vi "PID Autotune Y-Axis.vi"() -> ()   [LabVIEW 2017]
uses:
  <vilib>/addons/control/pid/autopid.llb/PID autotuning parameters (adv).ctl
  <vilib>/myRIO/Common/Instrument Driver Framework/myRIO v1.0/UART/vis/myRIO v1.0 Close UART.vi
  <vilib>/addons/control/pid/pid.llb/PID Control Input Filter (DBL).vi
  <vilib>/myRIO/Common/Instrument Driver Framework/Utilities/vis/FPGA Ref Manager.vi
  <vilib>/myRIO/Common/Instrument Driver Framework/myRIO v1.0/myRIO v1.0 Reset FPGA.vi
  <vilib>/myRIO/Common/Instrument Driver Framework/myRIO v1.0/IRQ/vis/myRIO v1.0 IRQ Info FGV.vi
  <vilib>/myRIO/Common/Instrument Driver Framework/myRIO v1.0/IRQ/vis/myRIO v1.0 Timer IRQ Info FGV.vi
  <vilib>/myRIO/Common/Instrument Driver Framework/myRIO v1.0/IRQ/vis/myRIO v1.0 ISR Agent.vi
  <vilib>/myRIO/Instrument Drivers/Utilities/Utilities.lvlib
  <vilib>/addons/control/pid/NI_PID_pid.lvlib
  <vilib>/addons/control/pid/NI_PID_autopid.lvlib
  <vilib>/ptbypt/NI_PtbyPt.lvlib
panel:
  in  "alpha":dbl=0.1 format="%.2f"
  in  "gamma":dbl format="%.2f"
  in  "autotuning parameters":T1={"technique"=2, "type of controller"=1, "control specification"=0, "amplitude"=1.0} {"amplitude" format="%.2f"; "control specification" items=["normal", "fast", "slow"]; "type of controller" items=["P", "PI", "PID"]; "technique" items=["Step Open Loop", "Step Closed Loop", "Relay", "PID Relay"]}
  in  "reinitialize? (F)":bool
  out "tuning completed?":bool
  in  "auto? (F)":bool
  out "tuned PID gains":T2={"proportional gain (Kc)"=1.0, "integral time (Ti, min)"=0.01, "derivative time (Td, min)"=0.0} {"derivative time (Td, min)" format="%#.6g"; "integral time (Ti, min)" format="%#.6g"; "proportional gain (Kc)" format="%#.6g"}
  in  "autotune? (F)":bool
  out "Sensor Output":cluster{dbl, "output":dbl}(graph)
  out "Motion Data":T3
  in  "FWD/RVS":bool
  out "Time (s)":dbl
  out "Output String":string
  out "PID Output":dbl(graph)
  out "SP & PV":T4(graph)
  in  "PID gains":T2={"proportional gain (Kc)"=1.0, "integral time (Ti, min)"=0.01, "derivative time (Td, min)"=0.0} {"derivative time (Td, min)" format="%.4f"; "integral time (Ti, min)" format="%.4f"; "proportional gain (Kc)" format="%.3f"}
  out "dt out (s)":dbl format="%.3f"
  in  "Velocity Set Pt":dbl
  in  "stop":bool
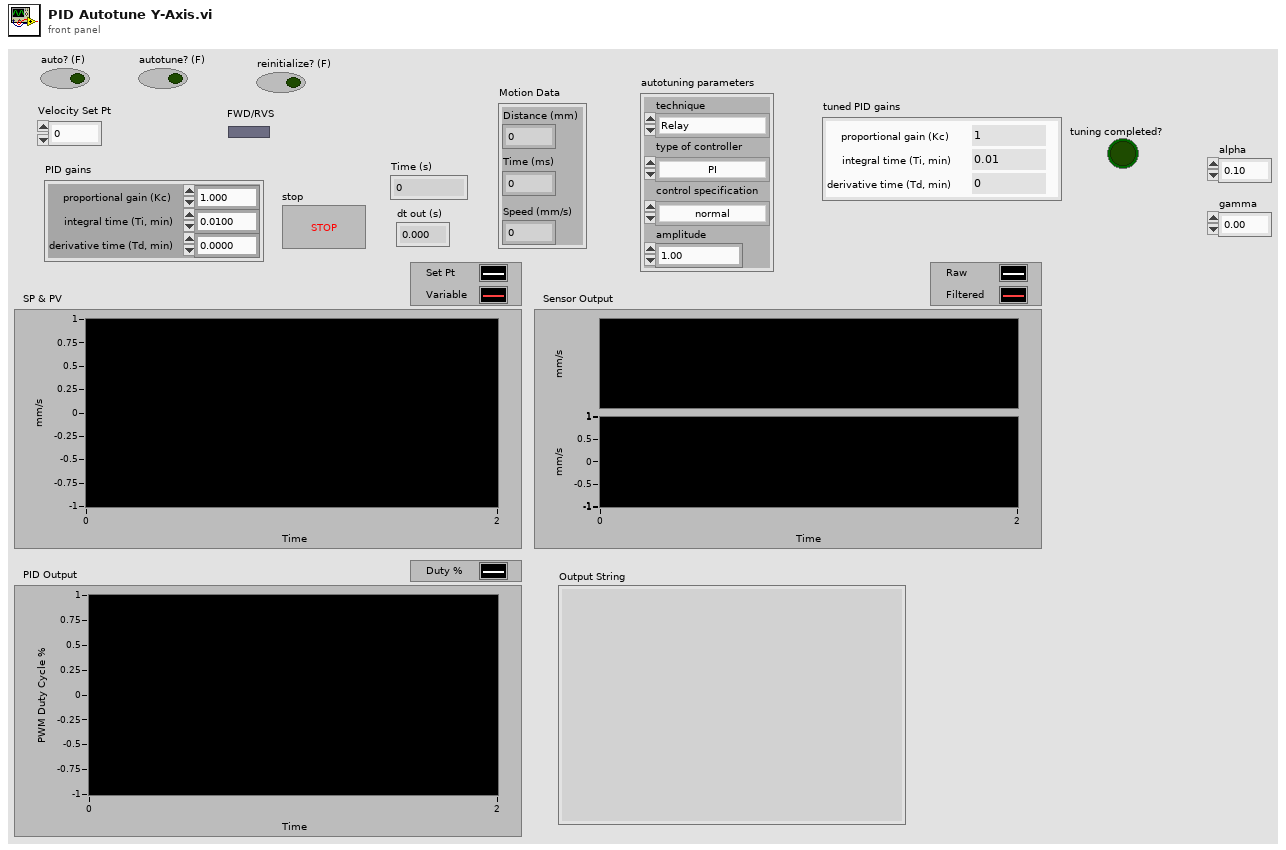
[diagram p1: front panel]
types:
  T1 = typedef "NI_PID_autopid.lvlib/PID autotuning parameters (adv).ctl" = cluster{"technique":u16, "type of controller":u16, "control specification":u16, "amplitude":dbl}
  T2 = cluster{"proportional gain (Kc)":dbl, "integral time (Ti, min)":dbl, "derivative time (Td, min)":dbl}
  T3 = cluster{"Distance (mm)":dbl, "Time (ms)":u32, "Speed (mm/s)":dbl}
  T4 = cluster{"Velocity Set Pt":dbl, "Velocity (mm/s)":dbl}
  T5 = cluster{"Velocity Set Pt":dbl, "Velocity (mm/s)":dbl}[]
  T6 = typedef "Encoder Cluster.ctl" = cluster{"Y-axis rev count":dbl, "Y-axis distance":dbl, "X-axis rev count":dbl, "X-axis distance":dbl, "Y-axis direction":T7, "X-axis direction":T7, "X-counter val":i32, "Y-counter val":i32}
  T7 = typedef "Encoder Count Direction Enum.ctl" = enum16{"Counting Up", "Counting Down"}
  T8 = cluster{dbl, "mean":dbl, "output":dbl, "output":dbl, "proportional gain (Kc)":dbl, "integral time (Ti, min)":dbl, "derivative time (Td, min)":dbl, dbl}
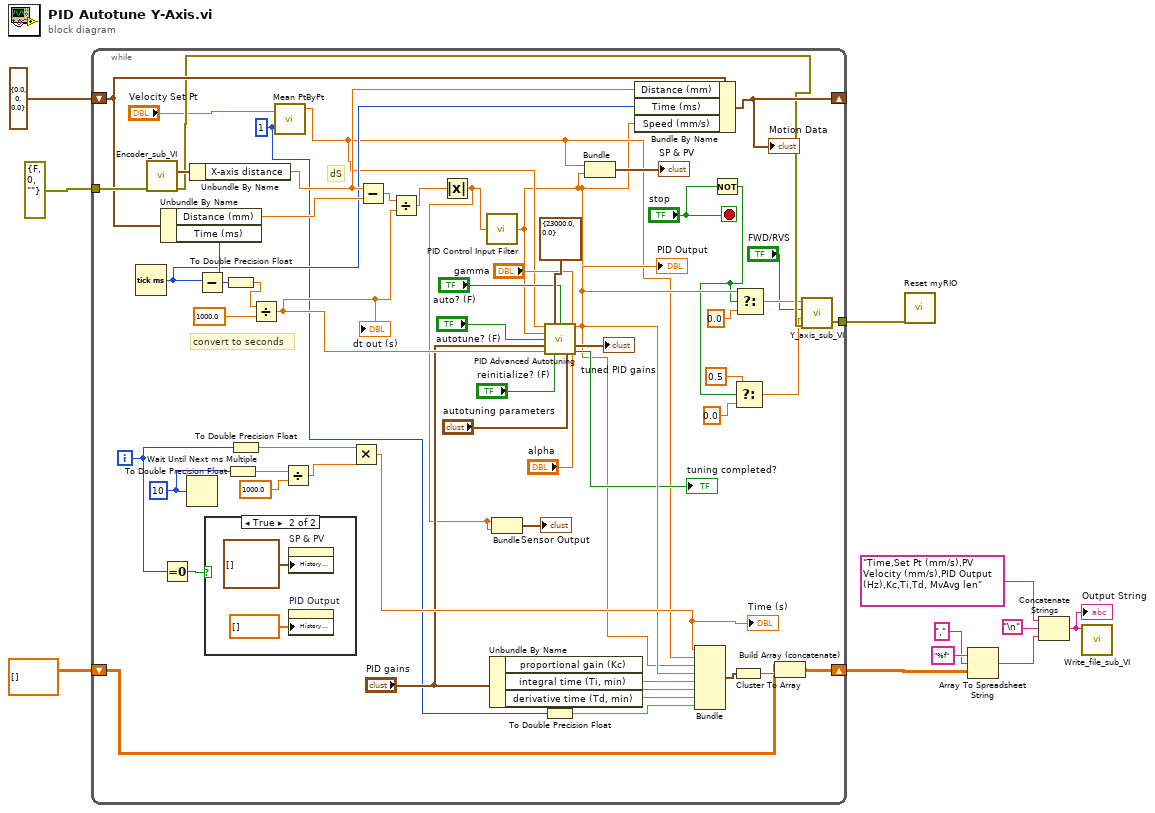
[diagram p0: block diagram]
diagram:
  n1 = while {
    shift-right: [w57] -> w4
    shift-left: dbl[][] [] ("element") -> [w58]
    tunnel: errorcluster {"status"=FALSE, "code"=0, "source"=""} ("error constant") -> [w56]
    tunnel: [w24] -> w2
    shift-right: [w39] -> _
    shift-left: T3 {"Distance (mm)"=0.0, "Time (ms)"=0, "Speed (mm/s)"=0.0} ("Motion Data") -> [w43]
    i -> [w45]
    stop <- "stop" stop-if-true
    w15 = 1 ("sample length")
    w47 = u32 10 ("millisecond multiple")
    # "dS"
    # "convert to seconds"
    n2 = Tick Count (ms)() -> (millisecond timer value=w40:u32)
    n3 = call "Encoder_sub_VI.vi"("error in (no error)"=w56) -> ("error out"=w25:errorcluster, "Encoder Output"=w69:T6)  [unwired: 9 in]
    n4 = Unbundle By Name(w43) -> ("Distance (mm)"=w44:dbl, "Time (ms)"=w41:u32)
    n5 = Equal To 0?(x=w45) -> (x = 0?=w46:bool)
    n6 = Wait Until Next ms Multiple(millisecond multiple=w47) -> ()  [unwired: 1 out]
    n7 = Unbundle By Name(w69) -> ("X-axis distance"=w42:dbl)
    n8 = Subtract(x=w40, y=w41) -> (x-y=w62:u32)
    n9 = case shown="True" w46 {
      frame False {
      }
      frame True {
        n10 = property on="SP & PV" class="WFChart (strict)"("History Data"=T5 []) -> ()  [unwired: 2 in, 2 out]
        n11 = property on="PID Output" class="WFChart (strict)"("History Data"=dbl[] []) -> ()  [unwired: 2 in, 2 out]
      }
    }
    n12 = To Double Precision Float(number=w62) -> (double precision float=w61:dbl)
    n13 = To Double Precision Float(number=w47) -> (double precision float=w55:dbl)
    n14 = To Double Precision Float(number=w45) -> (double precision float=w48:dbl)
    n15 = Divide(x=w61, y=1000.0) -> (x/y=w36:dbl)
    "dt out (s)" <- w36
    n16 = call <vilib>:"Mean PtByPt.vi"("x"="Velocity Set Pt", "sample length"=w15) -> ("mean"=w16:dbl)  [unwired: 2 in, 1 out]
    n17 = Divide(x=w55, y=1000.0) -> (x/y=w50:dbl)
    n18 = Multiply(x=w48, y=w50) -> (x*y=w49:dbl)
    "Time (s)" <- w49
    n19 = Subtract(x=w42, y=w44) -> (x-y=w67:dbl)
    n20 = Divide(x=w67, y=w36) -> (x/y=w66:dbl)
    n21 = Absolute Value(x=w66) -> (abs(x)=w13:dbl)
    n22 = call-poly <vilib>:"PID Control Input Filter.vi"("input"=w13) -> ("output"=w12:dbl)  [unwired: 4 in]
    n23 = Unbundle By Name("PID gains") -> ("proportional gain (Kc)"=w53:dbl, "integral time (Ti, min)"=w52:dbl, "derivative time (Td, min)"=w51:dbl)
    n24 = Bundle(w13, w13) -> (→"Sensor Output":cluster{dbl, dbl})  [unwired: 1 in]
    n25 = call <vilib>:"PID Advanced Autotuning.vi"("setpoint"=w16, "output range"=cluster{"output high":dbl, "output low":dbl} {"output high"=23000.0, "output low"=0.0}, "auto? (F)"="auto? (F)", "process variable"=w12, "gamma"="gamma", "autotune? (F)"="autotune? (F)", "alpha"="alpha", "PID gains"="PID gains", "dt (s)"=w36, "reinitialize? (F)"="reinitialize? (F)", "autotuning parameters"="autotuning parameters") -> ("output"=w33:dbl, "tuned PID gains"=→"tuned PID gains":T2, "tuning completed?"=→"tuning completed?":bool)  [unwired: 2 in]
    "PID Output" <- w33
    n26 = To Double Precision Float(number=w15) -> (double precision float=w14:dbl)
    n27 = Bundle("mean"=w16, "output"=w12) -> (→"SP & PV":cluster{"mean":dbl, "output":dbl})  [unwired: 1 in]
    n28 = Bundle By Name(cluster=w43, "Distance (mm)"=w42, "Time (ms)"=w40, "Speed (mm/s)"=w12) -> (w39:T3)
    "Motion Data" <- w39
    n29 = Bundle(w49, "mean"=w16, "output"=w12, "output"=w33, "proportional gain (Kc)"=w53, "integral time (Ti, min)"=w52, "derivative time (Td, min)"=w51, w14) -> (w60:T8)  [unwired: 1 in]
    n30 = Not(x="stop") -> (.not. x?=w20:bool)
    n31 = Cluster To Array(cluster=w60) -> (array=w59:dbl[])
    n32 = Select(t=0.5, s=w20, f=0.0) -> (s? t:f=w19:dbl)
    n33 = Select(t=w33, s=w20, f=0.0) -> (s? t:f=w23:dbl)
    n34 = Build Array (concatenate)(w58, w59) -> (w57:dbl[][])
    n35 = call "Y_axis_sub_VI.vi"("error in (no error)"=w25, "Duty Cycle"=w19, "FWD/RVS"="FWD/RVS", "Frequency"=w23) -> ("error out"=w24:errorcluster)  [unwired: 7 in]
  }
  n36 = call <vilib>:"Reset myRIO.vi"("error in (no error)"=w2) -> ()  [unwired: 10 in, 1 out]
  n37 = Array To Spreadsheet String(delimiter (Tab)=",", array=w4, 3:"%f" ("format string")) -> (spreadsheet string=w10:string)
  n38 = Concatenate Strings("Time,Set Pt (mm/s),PV Velocity (mm/s),PID Output (Hz),Kc,Ti,Td, MvAvg len", "\n", w10) -> (w9:string)
  "Output String" <- w9
  n39 = call "Write_file_sub_VI.vi"("Output String"=w9) -> ()  [unwired: 9 in, 2 out]
